vi "GetAnklePosEachCycle.vi"(8 "error in (no error)":errorcluster, 11 "Path":path) -> (0 "error out":errorcluster, 1 "VarColHeaders":string[](array[string]), 2 "JAEachCycle":dbl[][](array[numeric]), 3 "Path dup":path)   [LabVIEW 2016]
uses:
  CAlex2-Data/CAlex2_Data.lvclass
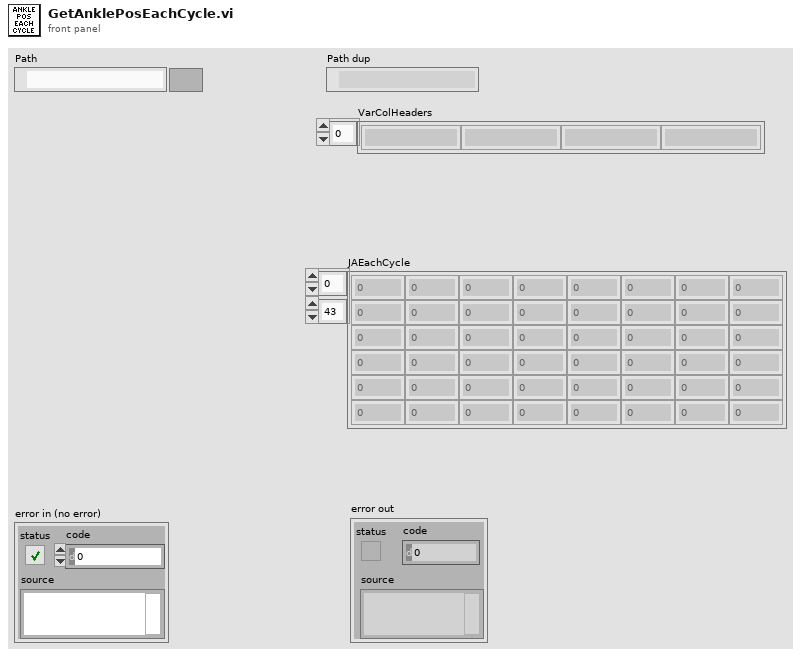
[diagram p1: front panel]
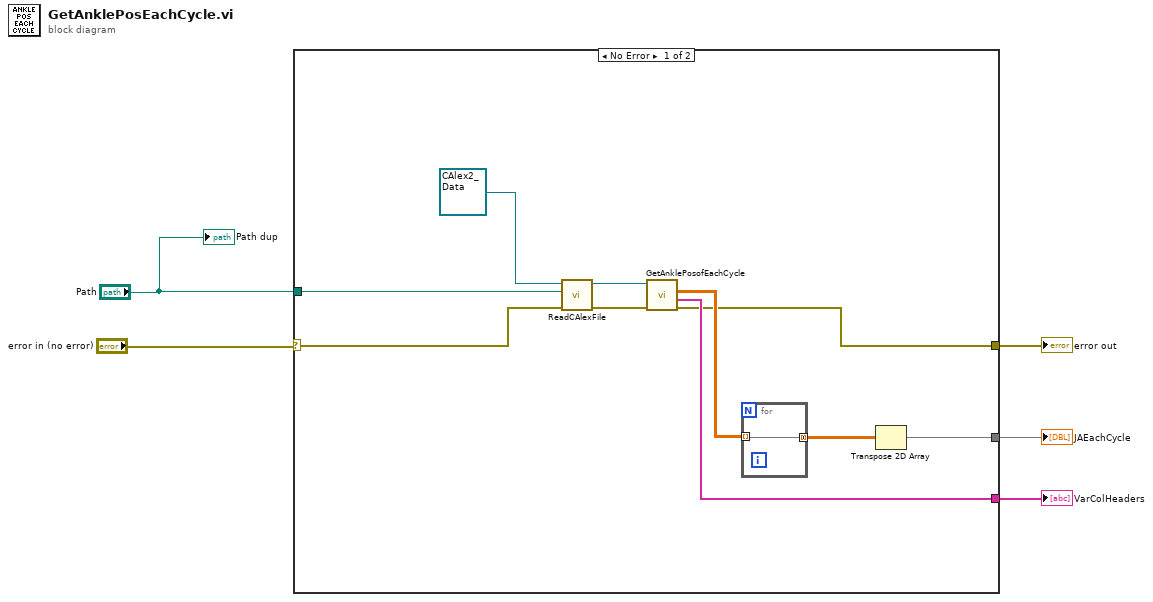
[diagram p0: block diagram]
diagram:
  n1 = case shown="No Error" "error in (no error)" {
    selector: "error in (no error)" -> [w11 w17]
    tunnel: "Path" -> [w15 _]
    tunnel: [w12 _] -> w5
    tunnel: [w6 w17] -> w4
    tunnel: [w7 _] -> w2
    frame No Error {
      n2 = call "ReadCAlexFile.vi"("error in (no error)"=w11, "ExpData File Path"=w15, "CAlexData2"=refnum<class "CAlex2_Data.lvclass"> refnum) -> ("error out"=w9:errorcluster, "CAlexData 2"=w10:refnum<class "CAlex2_Data.lvclass">)  [unwired: 7 in]
      n3 = call "GetAnklePosofEachCycle.vi"("error in (no error)"=w9, "CAlexData2 in"=w10) -> ("error out"=w6:errorcluster, "VarColHeaders"=w7:string[], "AnklePosEachCycle"=w8:dbl[][][])  [unwired: 6 in, 1 out]
      n4 = for {
        tunnel: w8 -> [w16] mode=indexing
        tunnel: [w16] -> w13 mode=concatenating
      }
      n5 = Transpose 2D Array(2D array=w13) -> (transposed array=w12:dbl[][])
    }
    frame Error {
    }
  }
  "error out" <- w4
  "JAEachCycle" <- w5
  "VarColHeaders" <- w2
  "Path dup" <- "Path"
